vi "Get Transactions by Date.vi"(8 "error in (no error)":errorcluster, 9 "Month":T1, 10 "YYYY":i32, 11 "Database in":refnum<class "Account History.lvclass">) -> (0 "error out":errorcluster, 1 "Credit Statement":refnum<class "Statement.lvclass">, 2 "Bank Statement":refnum<class "Statement.lvclass">, 3 "Database out":refnum<class "Account History.lvclass">)   [LabVIEW 2018, in "Account History.lvclass"]
uses:
  Account History.lvclass
  Statement/Statement.lvclass
  Month.ctl
  Banking Statement/Banking Statement.lvclass
  C:/Users/jtipps/Documents/Filthy-Lucre-Budgetizer/source/support/classes/Statement/Statement.lvclass
  Credit Statement/Credit Statement.lvclass
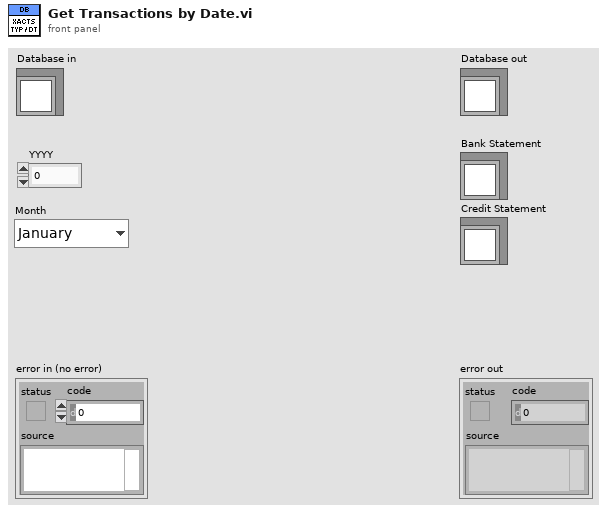
[diagram p1: front panel]
types:
  T1 = typedef "Account History.lvclass/Month.ctl" = enum16{"January", "February", "March", "April", "May", "June", "July", "August", "September", "October", "November", "December"}
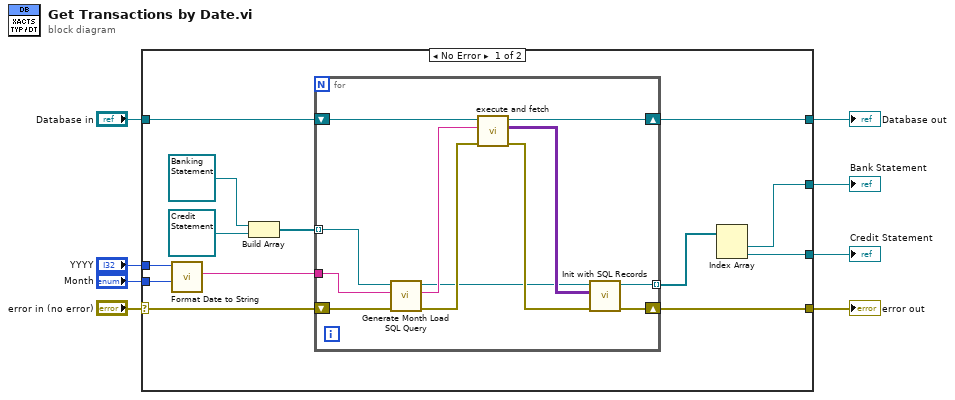
[diagram p0: block diagram]
diagram:
  n1 = case shown="No Error" "error in (no error)" {
    selector: "error in (no error)" -> [w18 w35]
    tunnel: [w19 w35] -> w7
    tunnel: [w20 w34] -> w5
    tunnel: "Database in" -> [w21 w34]
    tunnel: [w13 _] -> w4
    tunnel: [w12 _] -> w3
    tunnel: "YYYY" -> [w10 _]
    tunnel: "Month" -> [w9 _]
    frame No Error {
      n2 = call "Format Date to String.vi"("Month"=w9, "YYYY"=w10) -> ("Year-Mo"=w11:string)  [unwired: 9 in]
      n3 = Build Array(refnum<class "Banking Statement.lvclass"> refnum ("Banking Statement.lvclass"), refnum<class "Credit Statement.lvclass"> refnum ("Credit Statement.lvclass")) -> (w15:refnum<class "Statement.lvclass">[])
      n4 = for {
        tunnel: w11 -> [w25]
        shift-right: [w28] -> w20
        shift-left: w21 -> [w29]
        shift-right: [w27] -> w19
        shift-left: w18 -> [w26]
        tunnel: w15 -> [w24] mode=indexing
        tunnel: [w22] -> w14 mode=indexing
        n5 = call-dynamic "Generate Month Load SQL Query.vi"("error in (no error)"=w26, "Year-Mo"=w25, "Statement in"=w24) -> ("error out"=w31:errorcluster, "SQL Query"=w32:string, "Statement out"=w23:refnum<class "Statement.lvclass">)  [unwired: 6 in]
        n6 = call "execute and fetch.vi"("error in (no error)"=w31, "SQL query"=w32, "Database in"=w29) -> ("error out"=w30:errorcluster, "recordset data"=w33:variant[][], "Database out"=w28:refnum<class "Account History.lvclass">)  [unwired: 5 in, 1 out]
        n7 = call-dynamic "Init with SQL Records.vi"("error in (no error)"=w30, "SQL Dataset"=w33, "Statement in"=w23) -> ("error out"=w27:errorcluster, "Statement out"=w22:refnum<class "Statement.lvclass">)  [unwired: 7 in]
      }
      n8 = Index Array(array=w14) -> (element #1=w13:refnum<class "Statement.lvclass">, element #2=w12:refnum<class "Statement.lvclass">)  [unwired: 2 in]
    }
    frame Error {
    }
  }
  "error out" <- w7
  "Database out" <- w5
  "Bank Statement" <- w4
  "Credit Statement" <- w3
